vi "Compute Max Level.vi"(0 "Pulse Train in":refnum<class "Pulse Train.lvclass">, 1 "Filter in":refnum<class "Filter.lvclass">, 5 "Level in":refnum<class "Level.lvclass">, 7 "Fs (Hz)":dbl, 9 "Vmax":dbl, 11 "error in (no error)":errorcluster) -> (4 "Pulse Train out":refnum<class "Pulse Train.lvclass">, 6 "Level thru":refnum<class "Level.lvclass">, 10 "Lmax":dbl, 15 "error out":errorcluster)   [LabVIEW 2020, in "Pulse Train.lvclass"]
uses:
  Pulse Train.lvclass
  D:/Development/epl-vi-lib/Koop/KObject Class/KObject.lvclass
  Level/Level.lvclass
  Filter/Filter.lvclass
  Pulse Train.lvclass/Pulse Train.ctl
  Level/Level.lvclass/Level.ctl
  <vilib>/Analysis/2dsp.llb/Inverse Complex FFT.vi
  bcb57a5a-215e-4c33-8dbd-9eff76b037c0.vi
  Level/Read Fs.vi
  1eda625d-cbfb-4e4c-847e-a60ddaab0d2e.vi
  7134f5c9-b7d7-4780-98d4-1c4476315c22.vi
  aa152c71-1c1e-4541-ae35-8ed79230f965.vi
  Level/Read Level.vi
  Level/Read Optical.vi
  Level/Read Static.vi
  Level/Write multiplier.vi
  Level/Read Units.vi
  Koop/KObject Class/KObject.lvclass
  <vilib>/Analysis/NI_AALPro.lvlib
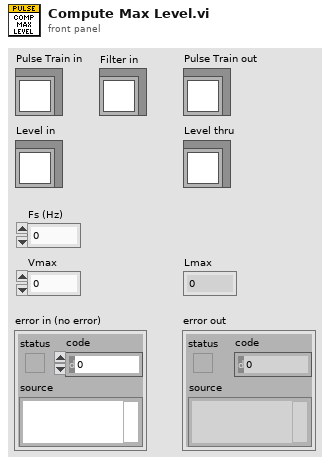
[diagram p1: front panel]
types:
  T1 = typedef "Level.lvclass/LevelUnits.ctl" = enum16{"dB atten", "dB SPL", "dB Vrms", "Volts", "dB mW", "mW", "dB HL", "dB SL"}
  T2 = cluster{"Freq (Hz)":dbl[], "Mag (dB SPL)":dbl[], "Phase (deg)":dbl[]}
  T3 = cluster{"Volts":dbl[], "Width":dbl[], "Rate":dbl[], "Power":dbl[][][][]}
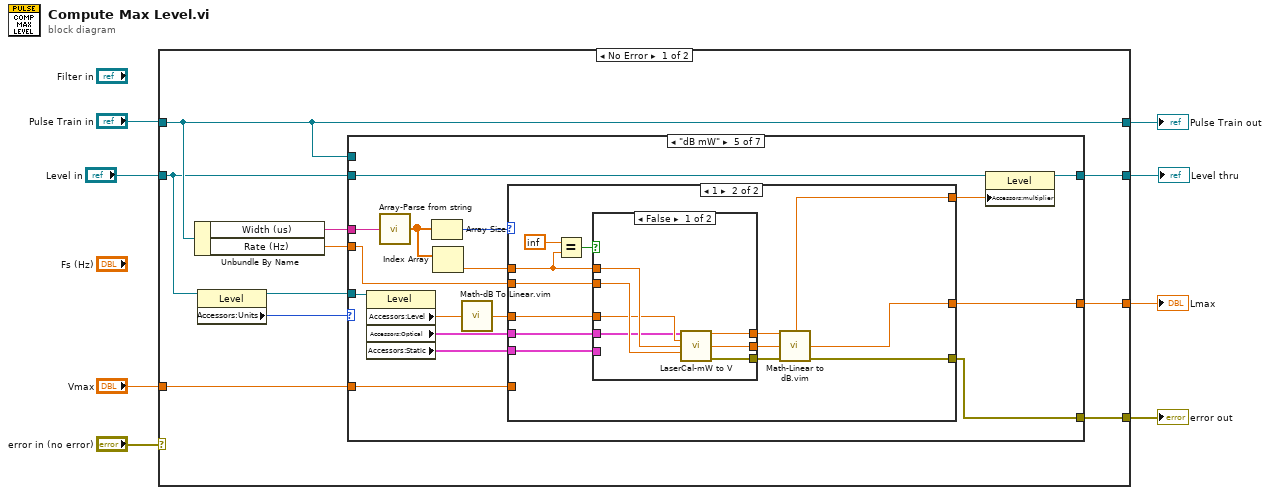
[diagram p0: block diagram]
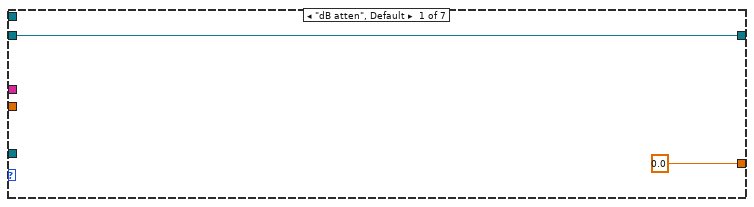
[diagram p2: hidden frame]
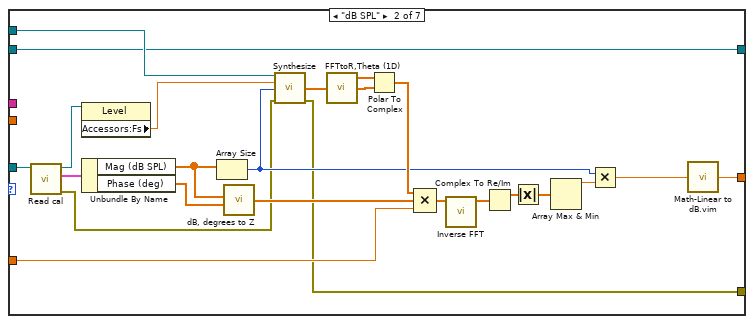
[diagram p3: hidden frame]
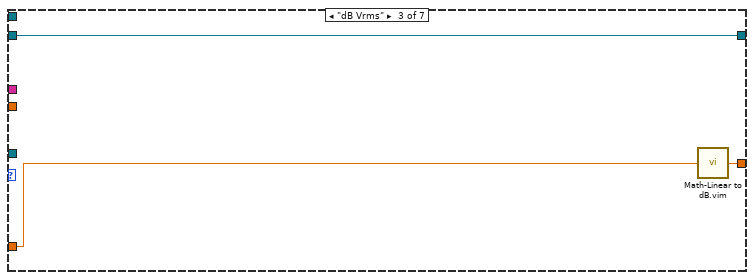
[diagram p4: hidden frame]
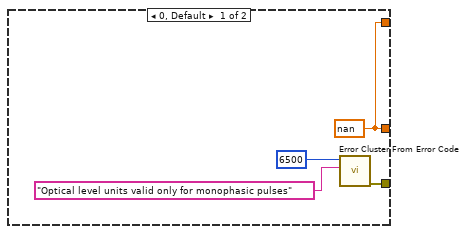
[diagram p6: hidden frame]
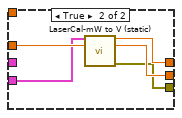
[diagram p7: hidden frame]
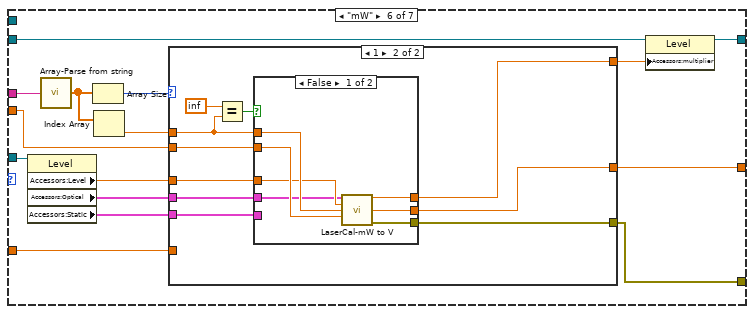
[diagram p8: hidden frame]
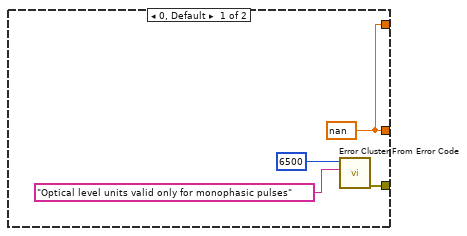
[diagram p9: hidden frame]
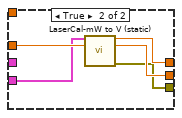
[diagram p10: hidden frame]
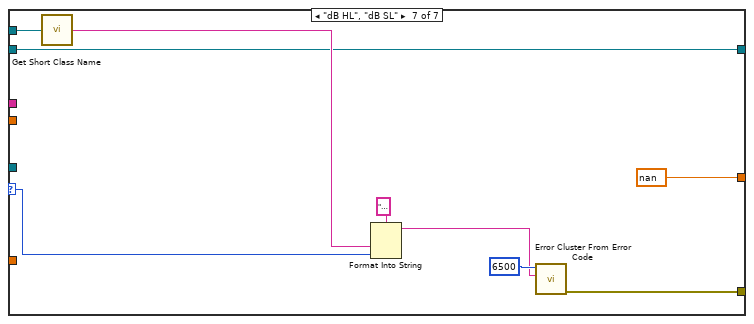
[diagram p11: hidden frame]
diagram:
  n1 = case shown="No Error" "error in (no error)" {
    selector: "error in (no error)" -> [_ w144]
    tunnel: "Pulse Train in" -> [w11 w145]
    tunnel: [w11 w145] -> w7
    tunnel: "Level in" -> [w10 w143]
    tunnel: "Vmax" -> [w15 _]
    tunnel: [w14 _] -> w2
    tunnel: [w13 w144] -> w4
    tunnel: [w9 w143] -> w1
    frame No Error {
      n2 = Unbundle By Name(w11) -> ("Width (us)"=w17:string, "Rate (Hz)"=w16:dbl)
      n3 = property class="Level"(reference=w10) -> (reference out=w12:refnum<class "Level.lvclass">, "Accessors:Units"=w18:T1)  [unwired: 1 in, 1 out]
      n4 = case shown="\"dB mW\"" w18 {
        selector: w18 -> [_ _ _ _ _ _ w137]
        tunnel: [0.0 ("Reference Level") w26 w47 w49 w53 w96 nan ("Vmax")] -> w14
        tunnel: [_ w22 _ _ w54 w97 w139] -> w13
        tunnel: w17 -> [_ _ _ _ w58 w101 _]
        tunnel: w16 -> [_ _ _ _ w63 w106 _]
        tunnel: w15 -> [_ w31 w46 w49 w64 w107 _]
        tunnel: w11 -> [_ w42 _ _ _ _ w136]
        tunnel: w12 -> [_ w44 _ _ w62 w105 _]
        tunnel: w10 -> [w19 w21 w45 w48 w52 w95 w134]
        tunnel: [w19 w21 w45 w48 w51 w94 w134] -> w9
        frame "dB atten", Default {
        }
        frame "dB SPL" {
          n5 = call "Read cal.vi"("Level in"=w44) -> ("error out"=w23:errorcluster, "cal"=w43:T2, "Level out"=w25:refnum<class "Level.lvclass">)  [unwired: 8 in]
          n6 = property class="Level"(reference=w25) -> ("Accessors:Fs"=w24:dbl)  [unwired: 1 in, 2 out]
          n7 = Unbundle By Name(w43) -> ("Mag (dB SPL)"=w32:dbl[], "Phase (deg)"=w33:dbl[])
          n8 = Array Size(array=w32) -> (size(s)=w27:i32)
          n9 = call "dB, degrees to Z.vi"("Magnitude (dB)"=w32, "Phase (degrees)"=w33) -> ("Z"=w34:cdb[])  [unwired: 5 in]
          n10 = call-dynamic "Synthesize.vi"("Pulse Train in"=w42, "Fs (Hz)"=w24, "Npts"=w27, "error in (no error)"=w23) -> ("Array"=w30:dbl[], "error out"=w22:errorcluster)  [unwired: 9 in, 1 out]
          n11 = call "FFTtoR,Theta (1D).VI"("X"=w30) -> ("+Freq. Mag of FFT"=w36:dbl[], "+Freq Theta of FFT"=w35:dbl[])  [unwired: 1 in]
          n12 = Polar To Complex(1:w35, 2:w36) -> (0:w29:cdb[])
          n13 = Compound Arithmetic op=MULTIPLY(w29, w34, w31) -> (w37:cdb[])
          n14 = call-poly <vilib>:"Inverse FFT.vi"("FFT {X}"=w37) -> ("X"=w38:cdb[])  [unwired: 9 in, 1 out]
          n15 = Complex To Re/Im(x + iy=w38) -> (x=w39:dbl[])  [unwired: 1 out]
          n16 = Absolute Value(x=w39) -> (abs(x)=w40:dbl[])
          n17 = Array Max & Min(array=w40) -> (max value=w28:dbl)  [unwired: 3 out]
          n18 = Multiply(x=w27, y=w28) -> (x*y=w41:dbl)
          n19 = call "Math-Linear to dB.vim"("linear"=w41) -> ("dB"=w26:dbl)
        }
        frame "dB Vrms" {
          n20 = call "Math-Linear to dB.vim"("linear"=w46) -> ("dB"=w47:dbl)
        }
        frame "Volts" {
        }
        frame "dB mW" {
          n21 = property class="Level"(reference=w62) -> ("Accessors:Level"=w61:dbl, "Accessors:Optical"=w60:T3, "Accessors:Static"=w59:cluster{"Voltage":dbl[], "Power":dbl[]})  [unwired: 1 in, 2 out]
          n22 = call "Array-Parse from string.vi"("String"=w58) -> ("Array"=w56:dbl[])  [unwired: 13 in, 1 out]
          n23 = Array Size(array=w56) -> (size(s)=w57:i32)
          n24 = Index Array(array=w56) -> (element=w55:dbl)  [unwired: 1 in]
          n25 = call "Math-dB To Linear.vim"("dB"=w61) -> ("linear"=w65:dbl)
          n26 = case shown="1" w57 {
            tunnel: w65 -> [_ w78]
            tunnel: w64 -> [_ _]
            tunnel: w63 -> [_ w76]
            tunnel: w60 -> [_ w75]
            tunnel: w59 -> [_ w74]
            tunnel: w55 -> [_ w73]
            tunnel: [w69 w72] -> w54
            tunnel: [w66 w71] -> w53
            tunnel: [w66 w70] -> w50
            frame 0, Default {
              w66 = nan ("dB")
              n27 = call <vilib>:"Error Cluster From Error Code.vi"("error message (\"\")"="Optical level units valid only for monophasic pulses", "error code (0)"=6500) -> ("error out"=w69:errorcluster)  [unwired: 7 in]
            }
            frame 1 {
              n28 = Equal?(x=inf, y=w73) -> (x = y?=w79:bool)
              n29 = case shown="False" w79 {
                tunnel: [w87 w90] -> w72
                tunnel: w76 -> [w86 _]
                tunnel: w73 -> [w85 _]
                tunnel: [w84 w91] -> w77
                tunnel: [w83 w92] -> w70
                tunnel: w78 -> [w82 w89]
                tunnel: w75 -> [w81 _]
                tunnel: w74 -> [_ w88]
                frame False {
                  n30 = call "LaserCal-mW to V.vi"("I-O"=w81, "Power (mW)"=w82, "Pulse width (us)"=w85, "Pulse rate (Hz)"=w86) -> ("Volts"=w83:dbl, "Max (mW)"=w84:dbl, "error out"=w87:errorcluster)  [unwired: 9 in]
                }
                frame True {
                  n31 = call "LaserCal-mW to V (static).vi"("I-O"=w88, "Level"=w89) -> ("Voltage"=w92:dbl, "Max Power"=w91:dbl, "error out"=w90:errorcluster)  [unwired: 11 in]
                }
              }
              n32 = call "Math-Linear to dB.vim"("linear"=w77) -> ("dB"=w71:dbl)
            }
          }
          n33 = property class="Level"(reference=w52, "Accessors:multiplier"=w50) -> (reference out=w51:refnum<class "Level.lvclass">)  [unwired: 1 in, 1 out]
        }
        frame "mW" {
          n34 = property class="Level"(reference=w105) -> ("Accessors:Level"=w104:dbl, "Accessors:Optical"=w103:T3, "Accessors:Static"=w102:cluster{"Voltage":dbl[], "Power":dbl[]})  [unwired: 1 in, 2 out]
          n35 = call "Array-Parse from string.vi"("String"=w101) -> ("Array"=w99:dbl[])  [unwired: 13 in, 1 out]
          n36 = Array Size(array=w99) -> (size(s)=w100:i32)
          n37 = Index Array(array=w99) -> (element=w98:dbl)  [unwired: 1 in]
          n38 = case shown="1" w100 {
            tunnel: w104 -> [_ w119]
            tunnel: w107 -> [_ _]
            tunnel: w106 -> [_ w117]
            tunnel: w103 -> [_ w116]
            tunnel: w102 -> [_ w115]
            tunnel: w98 -> [_ w114]
            tunnel: [w111 w113] -> w97
            tunnel: [w108 w118] -> w96
            tunnel: [w108 w112] -> w93
            frame 0, Default {
              w108 = nan ("Max Power")
              n39 = call <vilib>:"Error Cluster From Error Code.vi"("error message (\"\")"="Optical level units valid only for monophasic pulses", "error code (0)"=6500) -> ("error out"=w111:errorcluster)  [unwired: 7 in]
            }
            frame 1 {
              n40 = Equal?(x=inf, y=w114) -> (x = y?=w120:bool)
              n41 = case shown="False" w120 {
                tunnel: [w128 w131] -> w113
                tunnel: w117 -> [w127 _]
                tunnel: w114 -> [w126 _]
                tunnel: [w125 w132] -> w118
                tunnel: [w124 w133] -> w112
                tunnel: w119 -> [w123 w130]
                tunnel: w116 -> [w122 _]
                tunnel: w115 -> [_ w129]
                frame False {
                  n42 = call "LaserCal-mW to V.vi"("I-O"=w122, "Power (mW)"=w123, "Pulse width (us)"=w126, "Pulse rate (Hz)"=w127) -> ("Volts"=w124:dbl, "Max (mW)"=w125:dbl, "error out"=w128:errorcluster)  [unwired: 9 in]
                }
                frame True {
                  n43 = call "LaserCal-mW to V (static).vi"("I-O"=w129, "Level"=w130) -> ("Voltage"=w133:dbl, "Max Power"=w132:dbl, "error out"=w131:errorcluster)  [unwired: 11 in]
                }
              }
            }
          }
          n44 = property class="Level"(reference=w95, "Accessors:multiplier"=w93) -> (reference out=w94:refnum<class "Level.lvclass">)  [unwired: 1 in, 1 out]
        }
        frame "dB HL", "dB SL" {
          n45 = call "Get Short Class Name.vi"("KObject in"=w136) -> ("Class"=w135:string)  [unwired: 4 in]
          n46 = Format Into String(format string="%s: Cannot set level in '%s'", w135, w137) -> (resulting string=w140:string)  [unwired: 2 in, 1 out]
          n47 = call <vilib>:"Error Cluster From Error Code.vi"("error message (\"\")"=w140, "error code (0)"=6500) -> ("error out"=w139:errorcluster)  [unwired: 7 in]
        }
      }
    }
    frame Error {
    }
  }
  "error out" <- w4
  "Pulse Train out" <- w7
  "Level thru" <- w1
  "Lmax" <- w2
